vi "读取简单二进制文件.vi"() -> ()   [LabVIEW 2010]
panel:
  out "数据":cluster{i32, string, bool}
  in  "文件（使用对话框）":path
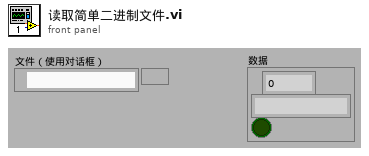
[diagram p1: front panel]
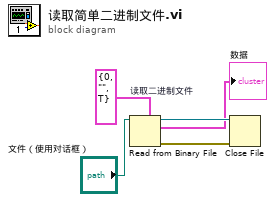
[diagram p0: block diagram]
diagram:
  n1 = Read from Binary File "读取二进制文件"(5:cluster{i32, string, bool} {0, "", TRUE}, 11:"文件（使用对话框）") -> (0:w4:errorcluster, 2:→"数据":cluster{i32, string, bool}, 3:w5:refnum<file>)  [unwired: 4 in, 1 out]
  n2 = Close File(refnum=w5, error in=w4) -> ()  [unwired: 2 out]
